vi "Set_Current.vi"(8 "error in (no error)":errorcluster caption="entrée d'erreur (pas d'erreur)", 10 "Current":dbl, 11 "Power_Supply (Default) en entrée":refnum<class "Power_Supply (Default).lvclass">) -> (0 "error out":errorcluster caption="sortie d'erreur", 3 "Power_Supply (Default) en sortie":refnum<class "Power_Supply (Default).lvclass">)   [LabVIEW 2020, in "Library Instrument & Equipement.lvlib" / "Library Power_Supply.lvlib" / "Power_Supply (Default).lvclass"]
uses:
  Power_Supply (Default).lvclass
  Power_Supply (Default).lvclass/Power_Supply (Default).ctl
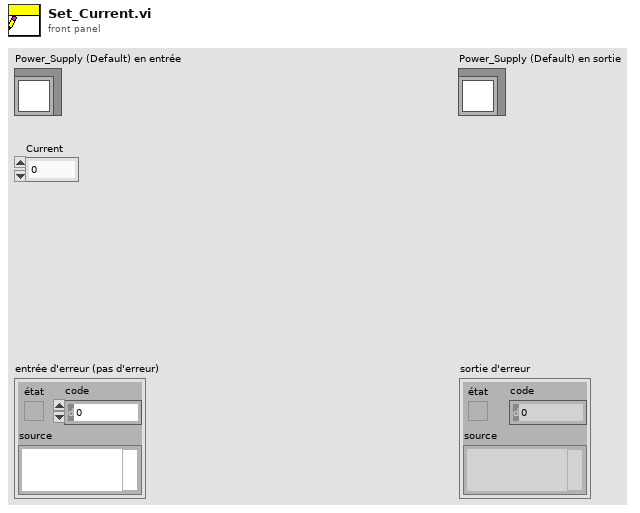
[diagram p1: front panel]
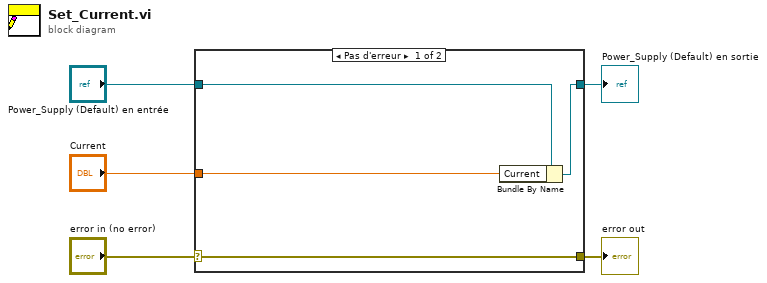
[diagram p0: block diagram]
diagram:
  n1 = case shown="Pas d'erreur" "error in (no error)" {
    selector: "error in (no error)" -> [w9 w10]
    tunnel: [w9 w10] -> w4
    tunnel: [w7 w11] -> w2
    tunnel: "Power_Supply (Default) en entrée" -> [w8 w11]
    tunnel: "Current" -> [w6 _]
    frame No Error {
      n2 = Bundle By Name(cluster=w8, "Current"=w6) -> (w7:refnum<class "Power_Supply (Default).lvclass">)
    }
    frame Error {
    }
  }
  "error out" <- w4
  "Power_Supply (Default) en sortie" <- w2
